vi "滤波参数.vi"(7 "滤波次数":u32=5, 8 "error in (no error)":errorcluster, 11 "x":dbl format="%0.2f") -> (0 "error out":errorcluster, 3 "mode":dbl caption="众数" format="%0.2f")   [LabVIEW 2016, in "斯坦道多参数.lvlib"]
uses:
  <vilib>/Analysis/baseanly.llb/Mean (DBL).vi
  <vilib>/Analysis/NI_AALBase.lvlib
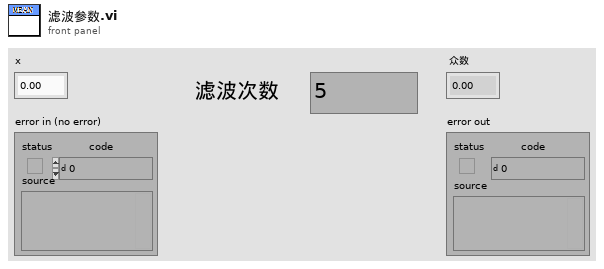
[diagram p1: front panel]
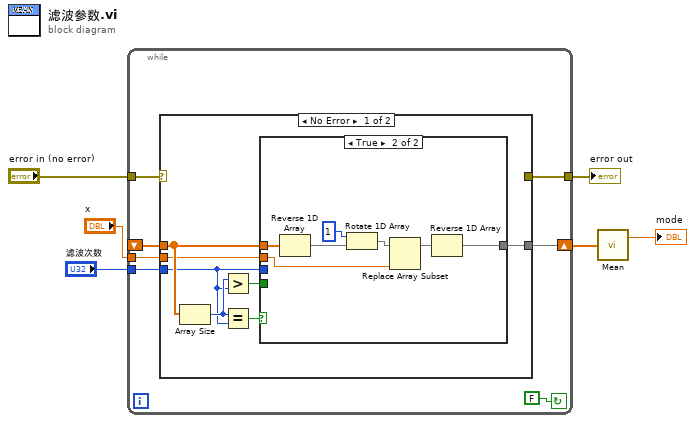
[diagram p0: block diagram]
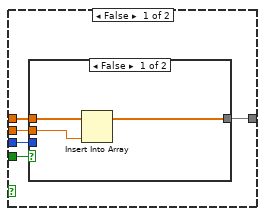
[diagram p2: hidden frame]
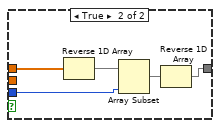
[diagram p3: hidden frame]
diagram:
  n1 = while {
    tunnel: "滤波次数" -> [w9]
    tunnel: "x" -> [w11]
    shift-right: [w10] -> w4
    shift-left: _ -> [w12]
    tunnel: "error in (no error)" -> [w8]
    tunnel: [w7] -> w1
    stop <- FALSE continue-if-true
    n2 = case shown="No Error" w8 {
      selector: w8 -> [_ w41]
      tunnel: w12 -> [w19 w42]
      tunnel: w11 -> [w18 _]
      tunnel: [w17 w42] -> w10
      tunnel: w9 -> [w14 _]
      tunnel: [_ w41] -> w7
      frame No Error {
        n3 = Array Size(array=w19) -> (size(s)=w16:i32)
        n4 = Greater?(x=w16, y=w14) -> (0:w15:bool)
        n5 = Equal?(x=w16, y=w14) -> (x = y?=w20:bool)
        n6 = case shown="True" w20 {
          tunnel: w19 -> [w25 w40]
          tunnel: w18 -> [w24 w38]
          tunnel: [w23 w34] -> w17
          tunnel: w15 -> [w22 _]
          tunnel: w14 -> [w21 _]
          frame False {
            n7 = case shown="False" w22 {
              tunnel: w25 -> [w28 w33]
              tunnel: w24 -> [w27 _]
              tunnel: [w26 w29] -> w23
              tunnel: w21 -> [_ w31]
              frame False {
                n8 = Insert Into Array(array=w28, new element=w27) -> (w26:dbl[])  [unwired: 1 in]
              }
              frame True {
                n9 = Reverse 1D Array(array=w33) -> (reversed array=w32:dbl[])
                n10 = Array Subset(array=w32, length=w31) -> (w30:dbl[])  [unwired: 1 in]
                n11 = Reverse 1D Array(array=w30) -> (reversed array=w29:dbl[])
              }
            }
          }
          frame True {
            n12 = Reverse 1D Array(array=w40) -> (reversed array=w35:dbl[])
            n13 = Rotate 1D Array(1:w35, 2:1 ("n")) -> (0:w39:dbl[])
            n14 = Replace Array Subset(array=w39, new element=w38) -> (w37:dbl[])  [unwired: 1 in]
            n15 = Reverse 1D Array(array=w37) -> (reversed array=w34:dbl[])
          }
        }
      }
      frame Error {
      }
    }
  }
  "error out" <- w1
  n16 = call-poly <vilib>:"Mean.vi"("X"=w4) -> ("mean"=→"mode":dbl)  [unwired: 1 out]
